vi "Create Digital Waveform.vi"(4 "error in":errorcluster, 5 "sample rate":dbl=1000.0, 6 "number of samples":u32, 7 "task in":refnum<k21>) -> (0 "error out":errorcluster, 2 "digital waveform array":digitalwaveform[](array[waveform]), 3 "task out":refnum<k21>)   [LabVIEW 2022 SP3]
doc: "This subVI creates an N dimensional Boolean array based on the number of channels in the task."
uses:
  <vilib>/Waveform/DWDTOps.llb/DWDT Boolean Array to Digital.vi
  <resource>/objmgr/daqmx.rc
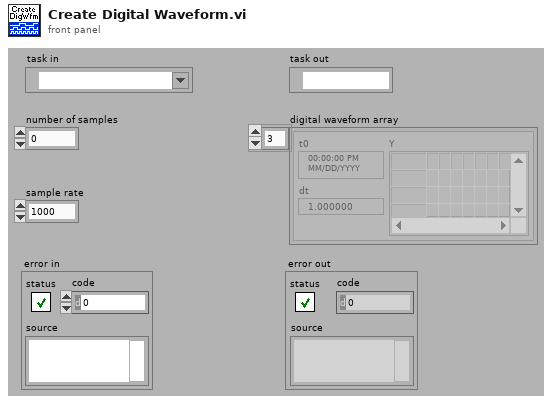
[diagram p1: front panel]
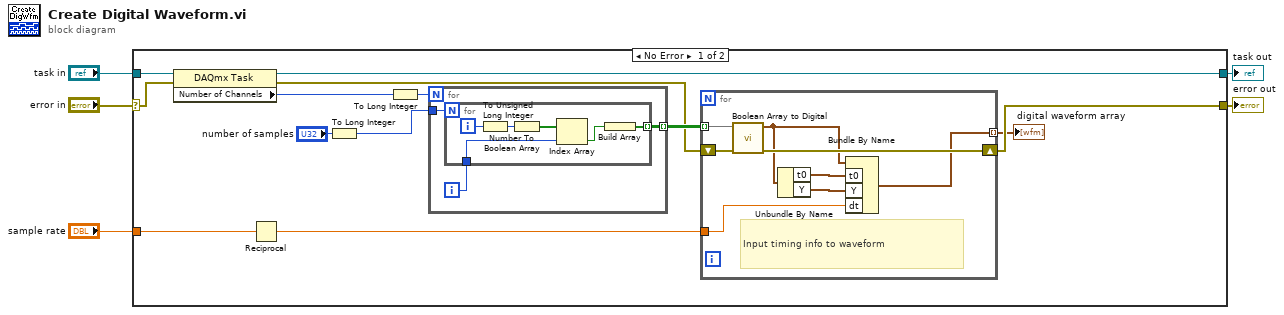
[diagram p0: block diagram]
diagram:
  n1 = case shown="No Error" "error in" {
    selector: "error in" -> [w10 w36]
    tunnel: "task in" -> [w16 w37]
    tunnel: [w15 w37] -> w4
    tunnel: [w14 w36] -> w2
    tunnel: "sample rate" -> [w7 _]
    frame No Error {
      n2 = property class="DAQmx Task"(reference=w16, error in=w10) -> (reference out=w15:refnum<k21>, error out=w17:errorcluster, "Number of Channels"=w12:u32)
      n3 = Reciprocal(x=w7) -> (1/x=w6:dbl)
      n4 = To Long Integer(number="number of samples") -> (32bit integer=w9:i32)
      n5 = To Long Integer(number=w12) -> (32bit integer=w8:i32)
      n6 = for {
        N: w8 -> [_]
        tunnel: [w29] -> w18 mode=indexing
        tunnel: w9 -> [w28]
        i -> [w27]
        n7 = for {
          N: w28 -> [_]
          tunnel: [w35] -> w29 mode=indexing
          tunnel: w27 -> [w30]
          i -> [w33]
          n8 = To Unsigned Long Integer(number=w33) -> (unsigned 32bit integer=w32:u32)
          n9 = Number To Boolean Array(number=w32) -> (Boolean array=w31:bool[])
          n10 = Index Array(array=w31, index=w30) -> (element=w34:bool)
          n11 = Build Array(w34) -> (w35:bool[])
        }
      }
      n12 = for {
        shift-right: [w26] -> w14
        shift-left: w17 -> [w25]
        tunnel: w18 -> [w24] mode=indexing
        tunnel: [w19] -> w13 mode=indexing
        tunnel: w6 -> [w21]
        # "Input timing info to waveform"
        n13 = call-poly <vilib>:"Boolean Array to Digital.vi"("error in (no error)"=w25, "boolean array"=w24) -> ("error out"=w26:errorcluster, "digital waveform"=w20:digitalwaveform)  [unwired: 8 in]
        n14 = Unbundle By Name(w20) -> ("t0"=w23:timestamp, "Y"=w22:digitaldata)
        n15 = Bundle By Name(cluster=w20, "t0"=w23, "Y"=w22, "dt"=w21) -> (w19:digitalwaveform)
      }
      "digital waveform array" <- w13
    }
    frame Error {
    }
  }
  "error out" <- w2
  "task out" <- w4
